vi "IRISS_FPGA_IO_v2.1.vi"() -> ()   [LabVIEW 2010]
doc: "This VI contains a basic quadrature decoder which is reset asynchronously upon clicking the reset button."
uses:
  <vilib>/platform/TimedLoop/XDataNode/XDataNode.xnode
  <vilib>/Platform/TimedLoop/XDataNode/nitl_modes.ctl
  <vilib>/Platform/TimedLoop/XDataNode/XDNodeRunTimeDep.lvlib
  <vilib>/Platform/TimedLoop/XDataNode/wakeup.ctl
  <vilib>/Platform/TimedLoop/XDataNode/timing_clust.ctl
  <vilib>/eio/EIONode/EIONode.xnode
  Library/KevinLibraryAll/labview/KevLib01.lvlib
  Library/jmslib.lvlib
panel:
  in  "Conn0/DIO15 Button 4":bool
  in  "Conn0/DIO12 Button 1":bool
  in  "Conn0/DIO13 Button 2":bool
  in  "Conn0/DIO14 Button 3":bool
  in  "DIR Y":bool
  in  "INHB Y":bool
  out "FAULT Y":bool
  out "Position Y":i32
  out "JumpBy2Error Y":i16
  in  "Reset Y":bool
  in  "Y DC":fxp<+,32,0>
  in  "DIR X":bool
  in  "INHB X":bool
  out "FAULT X":bool
  out "Position X":i32
  out "JumpBy2Error X":i16
  in  "Reset X":bool
  in  "DIR Z":bool
  in  "INHB Z":bool
  out "FAULTZ":bool
  out "Position Z":i32
  out "JumpBy2Error Z":i16
  in  "Reset Z":bool
  in  "Z DC":fxp<+,32,0>
  in  "X DC":fxp<+,32,0>
  out "samples":i32
  out "Current Monitor":u32[](array[numeric])
  out "Raw Data Response (MSB)":bool[](array[boolean])
  out "Home L4":bool
  out "Home L1":bool
  out "Home L2":bool
  out "Home L3":bool
  in  "Positive Direction C1-4":bool
  out "JumpBy2Error C1-4":i16
  out "32 bit Position C1-4":i32
  in  "Reset C1-4":bool
  in  "Positive Direction C1-1":bool
  out "JumpBy2Error C1-1":i16
  out "32 bit Position C1-1":i32
  in  "Reset C1-1":bool
  out "32 bit Position 17":i32
  in  "Reset 17":bool
  in  "Positive Direction 17":bool
  out "JumpBy2Error 17":i16
  out "32 bit Position 16":i32
  in  "Reset 16":bool
  in  "Positive Direction 16":bool
  out "JumpBy2Error 16":i16
  out "32 bit Position 15":i32
  in  "Reset 15":bool
  in  "Positive Direction 15":bool
  out "JumpBy2Error 15":i16
  out "32 bit Position 14":i32
  in  "Reset 14":bool
  in  "Positive Direction 14":bool
  out "JumpBy2Error 14":i16
  out "32 bit Position 13":i32
  in  "Reset 13":bool
  in  "Positive Direction 13":bool
  out "JumpBy2Error 13":i16
  out "32 bit Position 12":i32
  in  "Reset 12":bool
  in  "Positive Direction 12":bool
  out "JumpBy2Error 12":i16
  out "32 bit Position 11":i32
  in  "Reset 11":bool
  in  "Positive Direction 11":bool
  out "JumpBy2Error 11":i16
  out "32 bit Position 10":i32
  in  "Reset 10":bool
  in  "Positive Direction 10":bool
  out "JumpBy2Error 10":i16
  out "32 bit Position 9":i32
  in  "Reset 9":bool
  in  "Positive Direction 9":bool
  out "JumpBy2Error 9":i16
  out "JumpBy2Error 3":i16
  in  "Positive Direction 3":bool
  out "JumpBy2Error 1":i16
  in  "Positive Direction 1":bool
  out "AI":i16[](array[numeric])
  out "32 bit Position 3":i32
  in  "Reset 3":bool
  in  "AO":i16[](array[numeric])=[0, 0, 0, 0, 0, 0, 0, 0]
  out "32 bit Position 1":i32
  in  "Reset 1":bool
  # "Accurus Buttons"
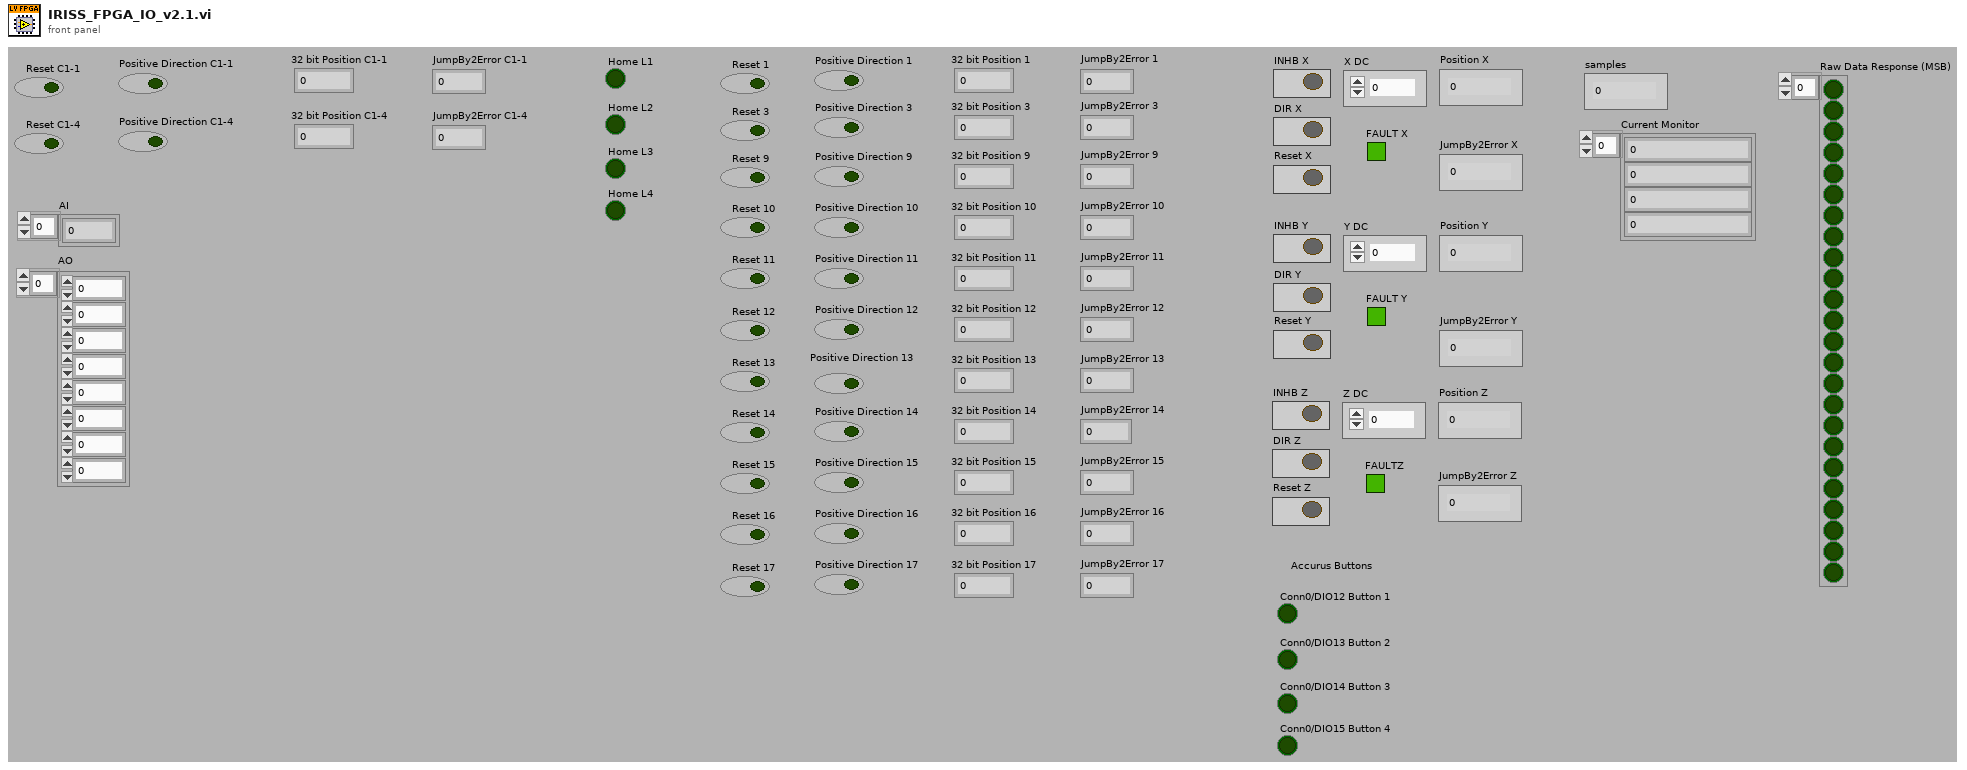
[diagram p1: front panel]
types:
  T1 = typedef "XDNodeRunTimeDep.lvlib/timing_clust.ctl" = cluster{"Expected End [f-1]":u64, "Actual End [f-1]":u64, "Finished Late? [f-1]":bool, "Expected End [i-1]":u64, "Actual End [i-1]":u64, "Finished Late? [i-1]":bool, "Expected Start [i]":u64, "Actual Start [i]":u64, "Expected Start [f]":u64, "Actual Start [f]":u64, "Source Name":string, "Structure Name":string, "Period":i64, "Deadline":i64, "Offset":i64, "Start":i64, "Priority":i32, "Timeout":i32, "Mode":T2, "Wakeup Reason":T3, "Error":errorcluster, "Source Type":string, "Secondary Source Type":string, "Global End Time":u64, "Global Start Time":u64, "Frame Duration":u64, "Iteration Duration":u64, "Assigned CPU":i32, "I/O Scan Engine Mode":u32}
  T2 = typedef "XDNodeRunTimeDep.lvlib/nitl_modes.ctl" = enum32{"No Change", "Process missed periods, maintain original phase", "Discard missed periods, maintain original phase", "Process missed periods, ignore original phase", "Discard missed periods, ignore original phase"}
  T3 = typedef "XDNodeRunTimeDep.lvlib/wakeup.ctl" = enum32{"Normal", "Aborted", "Asynchronous wakeup", "Timing source error", "Timed loop error", "Timeout"}
  T4 = cluster{"PWM In":refnum<k21>, "Direction":refnum<k21>, "Inhibit":refnum<k21>, "Encoder C":refnum<k21>, "Encoder B":refnum<k21>, "Encoder A":refnum<k21>, "Fault":refnum<k21>}
  T5 = cluster{"SCLK":refnum<k21>, "MOSI":refnum<k21>, "MISO":refnum<k21>}
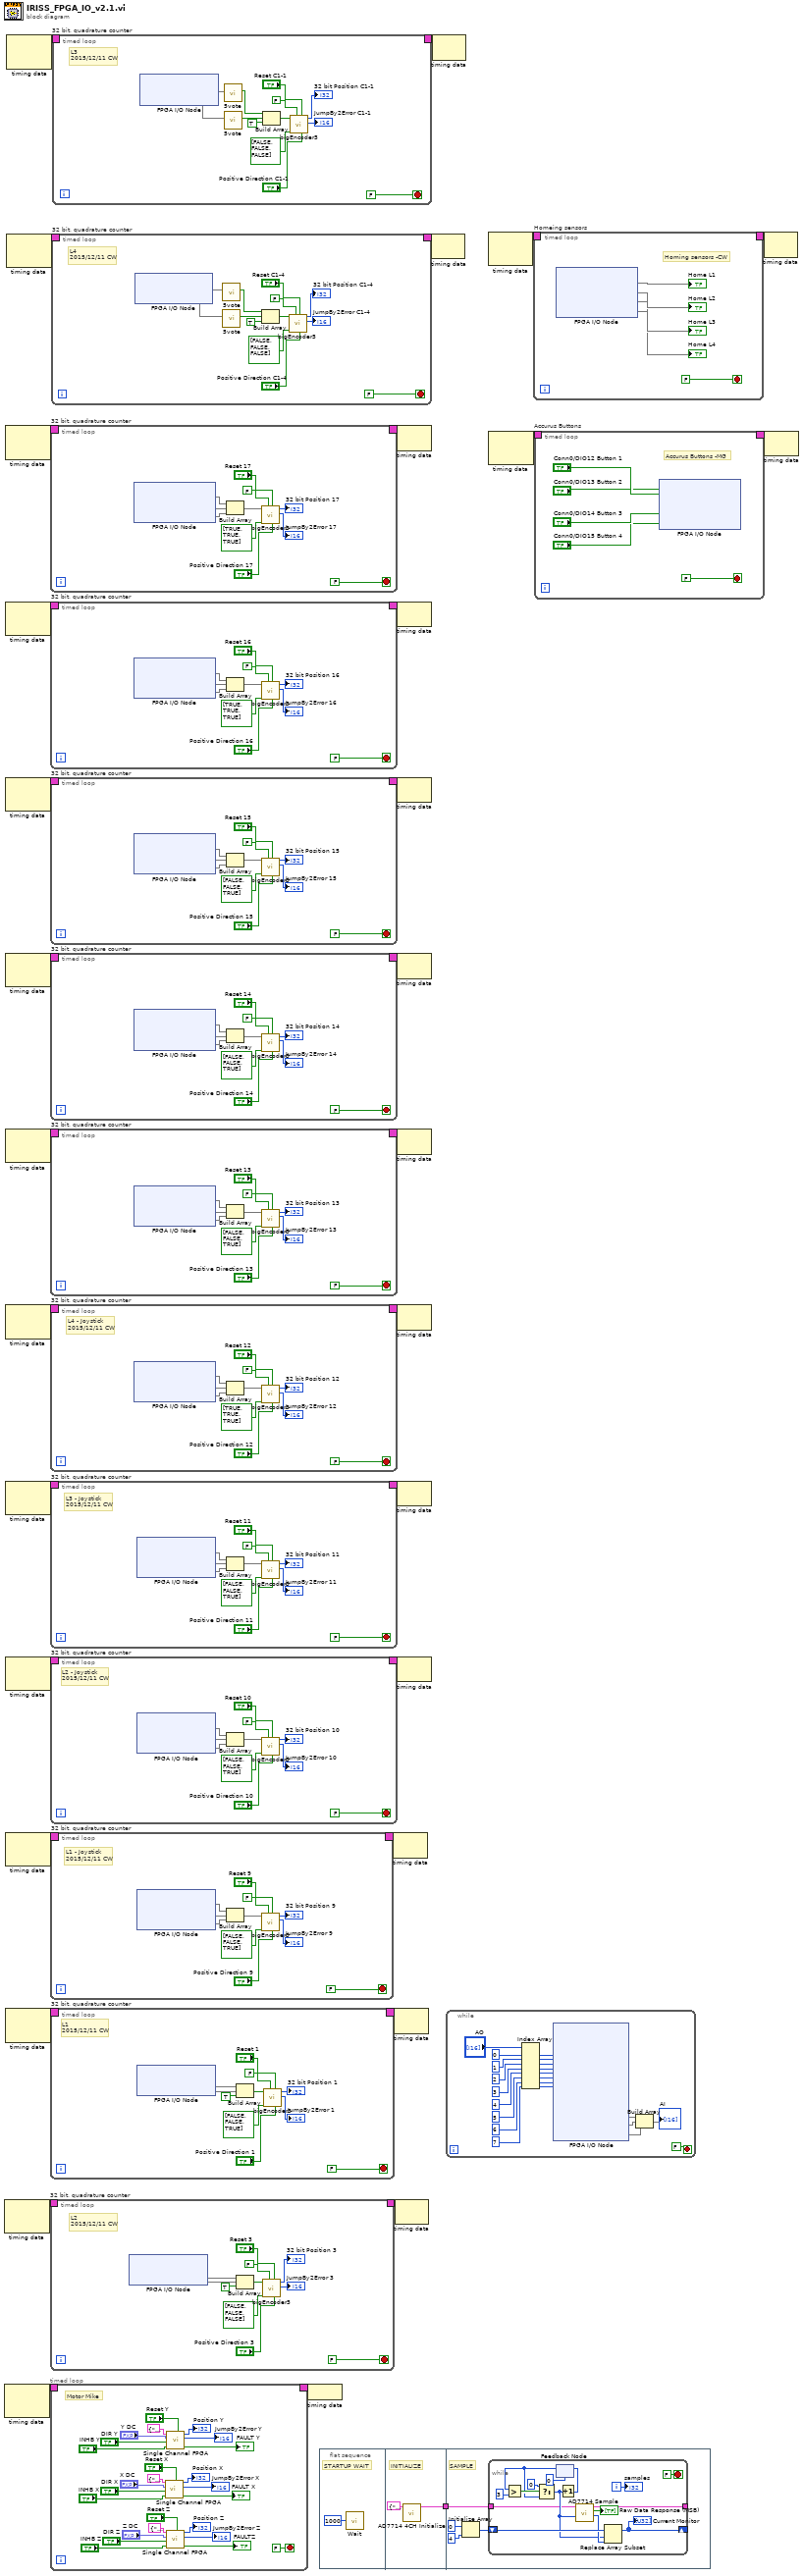
[diagram p0: block diagram]
diagram:
  n1 = node-c288() -> (w31:T1)  [unwired: 2 out]
  n2 = node-c288() -> (w5:T1)  [unwired: 2 in]
  n3 = node-c288() -> (w13:T1)  [unwired: 2 out]
  n4 = node-c288() -> (w15:T1)  [unwired: 2 out]
  n5 = node-c288() -> (w17:T1)  [unwired: 2 out]
  n6 = node-c288() -> (w19:T1)  [unwired: 2 out]
  n7 = node-c288() -> (w21:T1)  [unwired: 2 out]
  n8 = node-c288() -> (w23:T1)  [unwired: 2 out]
  n9 = node-c288() -> (w25:T1)  [unwired: 2 out]
  n10 = node-c288() -> (w27:T1)  [unwired: 2 out]
  n11 = node-c288() -> (w29:T1)  [unwired: 2 out]
  n12 = node-c288() -> (w32:T1)  [unwired: 2 out]
  n13 = node-c288() -> (w9:T1)  [unwired: 2 out]
  n14 = node-c288() -> (w11:T1)  [unwired: 2 out]
  n15 = timed-loop "32 bit, quadrature counter" {
    timing-out: [_] -> w30
    timing: w31 -> [_]
    stop <- FALSE stop-if-true
    # "L2\n2015/12/11 CW"
    n16 = xnode "FPGA I/O Node"() -> ("Connector0/DIO2"=w37, "Connector0/DIO3"=w36)  [unwired: 2 in, 2 out]
    n17 = Build Array(w37, w36, TRUE ("element")) -> (w43:bool[])
    n18 = call "bigEncoder3.vi"("Positive Direction"="Positive Direction 3", "ForceReset"="Reset 3", "Allow C Reset?"=FALSE, "Reset Array"=bool[] [FALSE, FALSE, FALSE], "Encoder Array"=w43) -> ("JumpBy2Error"=→"JumpBy2Error 3":i16, "Position"=→"32 bit Position 3":i32)  [unwired: 5 out]
  }
  n19 = timed-loop {
    timing: w5 -> [_]
    timing-out: [_] -> w4
    stop <- FALSE stop-if-true
    # "Motor Mike"
    n20 = call "Single Channel FPGA.vi"("Reset"="Reset X", "INHB"="INHB X", "DIR"="DIR X", "Duty"="X DC", "IO Channels"=T4 {"PWM In"="Connector1/DIO20", "Direction"="Connector1/DIO21", "Inhibit"="Connector1/DIO22", "Encoder C"="Connector1/DIO23", "Encoder B"="Connector1/DIO24", "Encoder A"="Connector1/DIO25", "Fault"="Connector1/DIO27"}) -> ("FAULT"=→"FAULT X":bool, "JumpBy2Error"=→"JumpBy2Error X":i16, "Position"=→"Position X":i32)  [unwired: 4 in]
    n21 = call "Single Channel FPGA.vi"("Reset"="Reset Z", "INHB"="INHB Z", "DIR"="DIR Z", "Duty"="Z DC", "IO Channels"=T4 {"PWM In"="Connector1/DIO14", "Direction"="Connector1/DIO15", "Inhibit"="Connector1/DIO16", "Encoder C"="Connector1/DIO17", "Encoder B"="Connector1/DIO18", "Encoder A"="Connector1/DIO19", "Fault"="Connector1/DIO26"}) -> ("FAULT"=→"FAULTZ":bool, "JumpBy2Error"=→"JumpBy2Error Z":i16, "Position"=→"Position Z":i32)  [unwired: 4 in]
    n22 = call "Single Channel FPGA.vi"("Reset"="Reset Y", "INHB"="INHB Y", "DIR"="DIR Y", "Duty"="Y DC", "IO Channels"=T4 {"PWM In"="Connector1/DIO1", "Direction"="Connector1/DIO2", "Inhibit"="Connector1/DIO3", "Encoder C"="Connector1/DIO4", "Encoder B"="Connector1/DIO5", "Encoder A"="Connector1/DIO6", "Fault"="Connector1/DIO0"}) -> ("FAULT"=→"FAULT Y":bool, "JumpBy2Error"=→"JumpBy2Error Y":i16, "Position"=→"Position Y":i32)  [unwired: 4 in]
  }
  n23 = timed-loop "32 bit, quadrature counter" {
    timing-out: [_] -> w12
    timing: w13 -> [_]
    stop <- FALSE stop-if-true
    n24 = xnode "FPGA I/O Node"() -> ("Connector2/DIO24"=w83, "Connector2/DIO25"=w82, "Connector2/DIO26"=w74)  [unwired: 3 in, 3 out]
    n25 = Build Array(w83, w82, w74) -> (w81:void[])
    n26 = call "bigEncoder3.vi"("Positive Direction"="Positive Direction 17", "ForceReset"="Reset 17", "Allow C Reset?"=FALSE, "Reset Array"=bool[] [TRUE, TRUE, TRUE], "Encoder Array"=w81) -> ("JumpBy2Error"=→"JumpBy2Error 17":i16, "Position"=→"32 bit Position 17":i32)  [unwired: 5 out]
  }
  n27 = timed-loop "32 bit, quadrature counter" {
    timing-out: [_] -> w14
    timing: w15 -> [_]
    stop <- FALSE stop-if-true
    n28 = xnode "FPGA I/O Node"() -> ("Connector2/DIO21"=w96, "Connector2/DIO22"=w95, "Connector2/DIO23"=w87)  [unwired: 3 in, 3 out]
    n29 = Build Array(w96, w95, w87) -> (w94:void[])
    n30 = call "bigEncoder3.vi"("Positive Direction"="Positive Direction 16", "ForceReset"="Reset 16", "Allow C Reset?"=FALSE, "Reset Array"=bool[] [TRUE, TRUE, TRUE], "Encoder Array"=w94) -> ("JumpBy2Error"=→"JumpBy2Error 16":i16, "Position"=→"32 bit Position 16":i32)  [unwired: 5 out]
  }
  n31 = timed-loop "32 bit, quadrature counter" {
    timing-out: [_] -> w16
    timing: w17 -> [_]
    stop <- FALSE stop-if-true
    n32 = xnode "FPGA I/O Node"() -> ("Connector2/DIO18"=w109, "Connector2/DIO19"=w108, "Connector2/DIO20"=w100)  [unwired: 3 in, 3 out]
    n33 = Build Array(w109, w108, w100) -> (w107:void[])
    n34 = call "bigEncoder3.vi"("Positive Direction"="Positive Direction 15", "ForceReset"="Reset 15", "Allow C Reset?"=FALSE, "Reset Array"=bool[] [FALSE, FALSE, TRUE], "Encoder Array"=w107) -> ("JumpBy2Error"=→"JumpBy2Error 15":i16, "Position"=→"32 bit Position 15":i32)  [unwired: 5 out]
  }
  n35 = timed-loop "32 bit, quadrature counter" {
    timing-out: [_] -> w18
    timing: w19 -> [_]
    stop <- FALSE stop-if-true
    n36 = xnode "FPGA I/O Node"() -> ("Connector2/DIO15"=w122, "Connector2/DIO16"=w121, "Connector2/DIO17"=w113)  [unwired: 3 in, 3 out]
    n37 = Build Array(w122, w121, w113) -> (w120:void[])
    n38 = call "bigEncoder3.vi"("Positive Direction"="Positive Direction 14", "ForceReset"="Reset 14", "Allow C Reset?"=FALSE, "Reset Array"=bool[] [FALSE, FALSE, TRUE], "Encoder Array"=w120) -> ("JumpBy2Error"=→"JumpBy2Error 14":i16, "Position"=→"32 bit Position 14":i32)  [unwired: 5 out]
  }
  n39 = timed-loop "32 bit, quadrature counter" {
    timing-out: [_] -> w20
    timing: w21 -> [_]
    stop <- FALSE stop-if-true
    n40 = xnode "FPGA I/O Node"() -> ("Connector2/DIO12"=w135, "Connector2/DIO13"=w134, "Connector2/DIO14"=w126)  [unwired: 3 in, 3 out]
    n41 = Build Array(w135, w134, w126) -> (w133:void[])
    n42 = call "bigEncoder3.vi"("Positive Direction"="Positive Direction 13", "ForceReset"="Reset 13", "Allow C Reset?"=FALSE, "Reset Array"=bool[] [FALSE, FALSE, TRUE], "Encoder Array"=w133) -> ("JumpBy2Error"=→"JumpBy2Error 13":i16, "Position"=→"32 bit Position 13":i32)  [unwired: 5 out]
  }
  n43 = timed-loop "32 bit, quadrature counter" {
    timing-out: [_] -> w22
    timing: w23 -> [_]
    stop <- FALSE stop-if-true
    # "L4 - Joystick\n2015/12/11 CW"
    n44 = xnode "FPGA I/O Node"() -> ("Connector2/DIO9"=w148, "Connector2/DIO10"=w147, "Connector2/DIO11"=w139)  [unwired: 3 in, 3 out]
    n45 = Build Array(w148, w147, w139) -> (w146:void[])
    n46 = call "bigEncoder3.vi"("Positive Direction"="Positive Direction 12", "ForceReset"="Reset 12", "Allow C Reset?"=FALSE, "Reset Array"=bool[] [TRUE, TRUE, TRUE], "Encoder Array"=w146) -> ("JumpBy2Error"=→"JumpBy2Error 12":i16, "Position"=→"32 bit Position 12":i32)  [unwired: 5 out]
  }
  n47 = timed-loop "32 bit, quadrature counter" {
    timing-out: [_] -> w24
    timing: w25 -> [_]
    stop <- FALSE stop-if-true
    # "L3 - Joystick\n2015/12/11 CW"
    n48 = xnode "FPGA I/O Node"() -> ("Connector2/DIO6"=w161, "Connector2/DIO7"=w160, "Connector2/DIO8"=w152)  [unwired: 3 in, 3 out]
    n49 = Build Array(w161, w160, w152) -> (w159:void[])
    n50 = call "bigEncoder3.vi"("Positive Direction"="Positive Direction 11", "ForceReset"="Reset 11", "Allow C Reset?"=FALSE, "Reset Array"=bool[] [FALSE, FALSE, TRUE], "Encoder Array"=w159) -> ("JumpBy2Error"=→"JumpBy2Error 11":i16, "Position"=→"32 bit Position 11":i32)  [unwired: 5 out]
  }
  n51 = timed-loop "32 bit, quadrature counter" {
    timing-out: [_] -> w26
    timing: w27 -> [_]
    stop <- FALSE stop-if-true
    # "L2 - Joystick\n2015/12/11 CW"
    n52 = xnode "FPGA I/O Node"() -> ("Connector2/DIO3"=w174, "Connector2/DIO4"=w173, "Connector2/DIO5"=w165)  [unwired: 3 in, 3 out]
    n53 = Build Array(w174, w173, w165) -> (w172:void[])
    n54 = call "bigEncoder3.vi"("Positive Direction"="Positive Direction 10", "ForceReset"="Reset 10", "Allow C Reset?"=FALSE, "Reset Array"=bool[] [FALSE, FALSE, TRUE], "Encoder Array"=w172) -> ("JumpBy2Error"=→"JumpBy2Error 10":i16, "Position"=→"32 bit Position 10":i32)  [unwired: 5 out]
  }
  n55 = timed-loop "32 bit, quadrature counter" {
    timing-out: [_] -> w28
    timing: w29 -> [_]
    stop <- FALSE stop-if-true
    # "L1 - Joystick\n2015/12/11 CW"
    n56 = xnode "FPGA I/O Node"() -> ("Connector2/DIO0"=w187, "Connector2/DIO1"=w186, "Connector2/DIO2"=w178)  [unwired: 3 in, 3 out]
    n57 = Build Array(w187, w186, w178) -> (w185:void[])
    n58 = call "bigEncoder3.vi"("Positive Direction"="Positive Direction 9", "ForceReset"="Reset 9", "Allow C Reset?"=FALSE, "Reset Array"=bool[] [FALSE, FALSE, TRUE], "Encoder Array"=w185) -> ("JumpBy2Error"=→"JumpBy2Error 9":i16, "Position"=→"32 bit Position 9":i32)  [unwired: 5 out]
  }
  n59 = timed-loop "32 bit, quadrature counter" {
    timing-out: [_] -> w33
    timing: w32 -> [_]
    stop <- FALSE stop-if-true
    # "L1\n2015/12/11 CW"
    n60 = xnode "FPGA I/O Node"() -> ("Connector0/DIO0"=w200, "Connector0/DIO1"=w199)  [unwired: 2 in, 2 out]
    n61 = Build Array(w200, w199, TRUE ("element")) -> (w198:bool[])
    n62 = call "bigEncoder3.vi"("Positive Direction"="Positive Direction 1", "ForceReset"="Reset 1", "Allow C Reset?"=FALSE, "Reset Array"=bool[] [FALSE, FALSE, TRUE], "Encoder Array"=w198) -> ("JumpBy2Error"=→"JumpBy2Error 1":i16, "Position"=→"32 bit Position 1":i32)  [unwired: 5 out]
  }
  n63 = timed-loop "32 bit, quadrature counter" {
    timing-out: [_] -> w8
    timing: w9 -> [_]
    stop <- FALSE stop-if-true
    # "L4\n2015/12/11 CW"
    n64 = xnode "FPGA I/O Node"() -> ("Connector0/DIO6"=w207, "Connector0/DIO7"=w206)  [unwired: 2 in, 2 out]
    n65 = call "5vote.vi"("Input"=w207) -> ("vote5"=w204:bool)  [unwired: 10 in]
    n66 = call "5vote.vi"("Input"=w206) -> ("vote5"=w205:bool)  [unwired: 10 in]
    n67 = Build Array(w204, w205, TRUE ("element")) -> (w215:bool[])
    n68 = call "bigEncoder3.vi"("Positive Direction"="Positive Direction C1-4", "ForceReset"="Reset C1-4", "Allow C Reset?"=FALSE, "Reset Array"=bool[] [FALSE, FALSE, FALSE], "Encoder Array"=w215) -> ("JumpBy2Error"=→"JumpBy2Error C1-4":i16, "Position"=→"32 bit Position C1-4":i32)  [unwired: 5 out]
  }
  n69 = timed-loop "32 bit, quadrature counter" {
    timing-out: [_] -> w10
    timing: w11 -> [_]
    stop <- FALSE stop-if-true
    # "L3\n2015/12/11 CW"
    n70 = xnode "FPGA I/O Node"() -> ("Connector0/DIO4"=w222, "Connector0/DIO5"=w221)  [unwired: 2 in, 2 out]
    n71 = call "5vote.vi"("Input"=w222) -> ("vote5"=w219:bool)  [unwired: 10 in]
    n72 = call "5vote.vi"("Input"=w221) -> ("vote5"=w220:bool)  [unwired: 10 in]
    n73 = Build Array(w219, w220, TRUE ("element")) -> (w230:bool[])
    n74 = call "bigEncoder3.vi"("Positive Direction"="Positive Direction C1-1", "ForceReset"="Reset C1-1", "Allow C Reset?"=FALSE, "Reset Array"=bool[] [FALSE, FALSE, FALSE], "Encoder Array"=w230) -> ("JumpBy2Error"=→"JumpBy2Error C1-1":i16, "Position"=→"32 bit Position C1-1":i32)  [unwired: 5 out]
  }
  n75 = node-c288(w4) -> ()
  n76 = flat-sequence {
    tunnel: [w235] -> w3
    tunnel: w3 -> [w237]
    frame #0 {
      # "STARTUP WAIT"
      n77 = call "Wait"("Count(uSec)"=u32 1000) -> ()  [unwired: 1 out]
    }
    frame #1 {
      # "INITIALIZE"
      n78 = call "AD7714 4CH Initialize.vi"("I/O Cluster In"=T5 {"SCLK"="Connector1/DIO29", "MOSI"="Connector1/DIO35", "MISO"="Connector1/DIO31"}) -> ("I/O Cluster Out"=w235:T5)  [unwired: 10 in]
    }
    frame #2 {
      # "SAMPLE"
      n79 = Initialize Array(u32 0, 4 ("dimension size")) -> (w238:u32[])
      n80 = while {
        shift-right: [w246] -> _
        shift-left: w238 -> [w247]
        tunnel: w237 -> [w243]
        tunnel: [w242] -> _
        i -> [w254]
        stop <- FALSE stop-if-true
        n81 = feedback #1(i16 0) -> (w250:i16)
        n82 = Greater?(x=w250, y=i16 3) -> (0:w251:bool)
        n83 = Select(t=i16 0, s=w251, f=w250) -> (s? t:f=w244:i16)
        n84 = Increment(x=w244) -> (x+1=w248:i16)
        n85 = feedback-in #1(w248) -> ()
        n86 = call "AD7714 Sample.vi"("Channel"=w244, "I/O Cluster In"=w243) -> ("Data"=w245:u32, "Raw Data Response (MSB)"=→"Raw Data Response (MSB)":bool[], "I/O Cluster Out"=w242:T5)  [unwired: 7 in]
        n87 = Replace Array Subset(array=w247, new element=w245, index=w244) -> (w246:u32[])
        "Current Monitor" <- w246
        "samples" <- w254
      }
    }
  }
  n88 = node-c288(w28) -> ()  [unwired: 1 out]
  n89 = node-c288(w33) -> ()  [unwired: 1 out]
  n90 = node-c288(w30) -> ()  [unwired: 1 out]
  n91 = node-c288(w12) -> ()  [unwired: 1 out]
  n92 = node-c288(w14) -> ()  [unwired: 1 out]
  n93 = node-c288(w16) -> ()  [unwired: 1 out]
  n94 = node-c288(w18) -> ()  [unwired: 1 out]
  n95 = node-c288(w20) -> ()  [unwired: 1 out]
  n96 = node-c288(w22) -> ()  [unwired: 1 out]
  n97 = node-c288(w24) -> ()  [unwired: 1 out]
  n98 = node-c288(w26) -> ()  [unwired: 1 out]
  n99 = node-c288(w8) -> ()  [unwired: 1 out]
  n100 = node-c288(w10) -> ()  [unwired: 1 out]
  n101 = while {
    stop <- FALSE stop-if-true
    n102 = Index Array(array="AO", index #1=0 ("index"), index #2=1 ("index"), index #3=2 ("index"), index #4=3 ("index"), index #5=4 ("index"), index #6=5 ("index"), index #7=6 ("index"), index #8=7 ("index")) -> (element #1=w268:i16, element #2=w267:i16, element #3=w266:i16, element #4=w265:i16, element #5=w264:i16, element #6=w263:i16, element #7=w262:i16, element #8=w261:i16)
    n103 = xnode "FPGA I/O Node"("Connector0/AO0"=w268, "Connector0/AO1"=w267, "Connector0/AO2"=w266, "Connector0/AO3"=w265, "Connector0/AO4"=w264, "Connector0/AO5"=w263, "Connector0/AO6"=w262, "Connector0/AO7"=w261) -> ("Connector0/AI0"=w259, "Connector0/AI1"=w258, "Connector0/AI2"=w256)  [unwired: 11 in, 11 out]
    n104 = Build Array(w259, w258, w256) -> (→"AI":void[])
  }
  n105 = node-c288() -> (w7:T1)  [unwired: 2 out]
  n106 = node-c288() -> (w2:T1)  [unwired: 2 out]
  n107 = timed-loop "Homeing sensors" {
    timing-out: [_] -> w6
    timing: w7 -> [_]
    stop <- FALSE stop-if-true
    # "Homing sensors -CW"
    n108 = xnode "FPGA I/O Node"() -> ("Connector0/DIO8"=→"Home L1", "Connector0/DIO9"=→"Home L2", "Connector0/DIO10"=→"Home L3", "Connector0/DIO11"=→"Home L4")  [unwired: 4 in, 4 out]
  }
  n109 = timed-loop "Accurus Buttons" {
    timing-out: [_] -> w1
    timing: w2 -> [_]
    stop <- FALSE stop-if-true
    # "Accurus Buttons -MG"
    n110 = xnode "FPGA I/O Node"("Connector0/DIO12"="Conn0/DIO12 Button 1", "Connector0/DIO13"="Conn0/DIO13 Button 2", "Connector0/DIO14"="Conn0/DIO14 Button 3", "Connector0/DIO15"="Conn0/DIO15 Button 4") -> ()  [unwired: 4 in, 4 out]
  }
  n111 = node-c288(w6) -> ()  [unwired: 1 out]
  n112 = node-c288(w1) -> ()  [unwired: 1 out]
